vi "Matrix_CommandsGlobal.vi"() -> ()   [LabVIEW 2019, in "Switching.lvclass"]
uses:
  Switching.lvclass
panel:
  in  "Matrix GPIB Setup":T1={"Matrix address"="", "Instrument name"="", "Instrument type"=2, "Command \"Matrix Reset\""="", "Command \"Connect Matrix Channels\""="", "Command \"Disconnect Matrix Channels\""=""} {"Instrument type" items=["Supply", "LCR", "Switching"]}
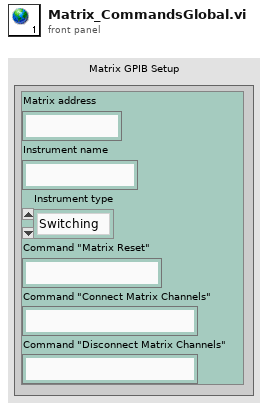
[diagram p1: front panel]
types:
  T1 = cluster{"Matrix address":string, "Instrument name":string, "Instrument type":u16, "Command \"Matrix Reset\"":string, "Command \"Connect Matrix Channels\"":string, "Command \"Disconnect Matrix Channels\"":string}
diagram:
